vi "_getInfoForWfmGeneration.vi"(11 "Analysis State":T1) -> (1 "wfm info":cluster{i32, "variant":variant}[](array[cluster]), 3 "number of channels":i32)   [LabVIEW 2017]
uses:
  <vilib>/addons/InsightCM/Utilities/Analysis/Shared/controls/AnalysisSensorType.ctl
  <vilib>/addons/InsightCM/Utilities/Analysis/Shared/controls/AnalysisConversionOp.ctl
  <vilib>/addons/InsightCM/Utilities/Analysis/Shared/controls/AnalysisBandDomain.ctl
  <vilib>/addons/InsightCM/Utilities/Analysis/Shared/controls/AnalysisFeature.ctl
  <vilib>/addons/InsightCM/Utilities/Analysis/Shared/controls/AnalysisDynamicChannel.ctl
  <vilib>/addons/InsightCM/Utilities/Analysis/Shared/controls/AnalysisCalculatedMeasurementType.ctl
  <vilib>/addons/InsightCM/Utilities/Analysis/Shared/controls/AnalysisBandAmplitudeScale.ctl
  <vilib>/addons/InsightCM/Utilities/Analysis/Shared/controls/AnalysisBandCalculation.ctl
  <vilib>/addons/InsightCM/Utilities/Analysis/Shared/controls/AnalysisStaticChannel.ctl
  <vilib>/addons/InsightCM/Utilities/Analysis/Shared/controls/AnalysisDevice.ctl
  <vilib>/addons/InsightCM/Utilities/Analysis/Shared/controls/AnalysisSpeedProfile.ctl
  <vilib>/addons/InsightCM/Utilities/Analysis/Shared/controls/AnalysisState.ctl
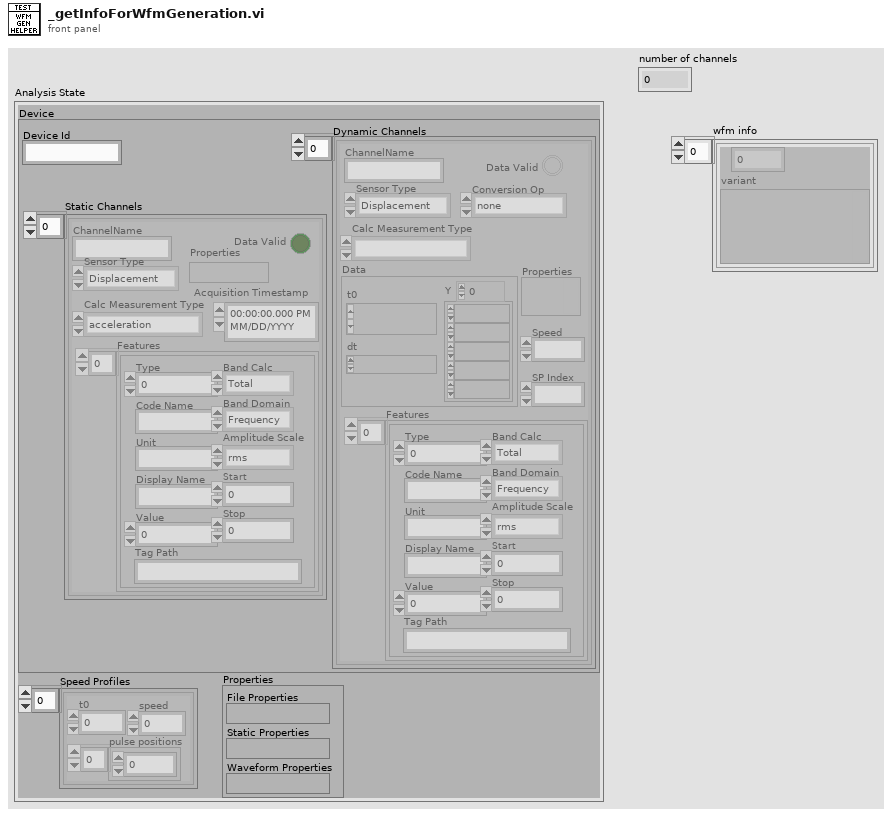
[diagram p1: front panel]
types:
  T1 = typedef "AnalysisState.ctl" = cluster{"Properties":cluster{"File Properties":variant, "Static Properties":variant, "Waveform Properties":variant}, "Properties Initialized?":bool, "Device":T2, "Speed Profiles":T12[]}
  T2 = typedef "AnalysisDevice.ctl" = cluster{"Device Id":string, "Dynamic Channels":T3[], "Static Channels":T11[]}
  T3 = typedef "AnalysisDynamicChannel.ctl" = cluster{"ChannelName":string, "Sensor Type":T4, "Conversion Op":T5, "Features":T6[], "Data":waveform(sgl), "Speed":sgl, "SP Index":i32, "Properties":variant, "Data Valid":bool, "Calc Measurement Type":T10}
  T4 = typedef "AnalysisSensorType.ctl" = enum16{"Accelerometer", "Velocity", "Displacement", "Tachometer", "Tempertature ", "dynamicVoltage", "Voltage", "Current", "Microphone", "Resistance", "Digital Input", "<Unknown>"}
  T5 = typedef "AnalysisConversionOp.ctl" = enum16{"none", "singleInt", "doubleInt", "singleDiff", "doubleDiff"}
  T6 = typedef "AnalysisFeature.ctl" = cluster{"Type":i32, "Code Name":string, "Unit":string, "Display Name":string, "Value":sgl, "Start":dbl, "Stop":dbl, "Band Domain":T7, "Band Calc":T8, "Amplitude Scale":T9, "Tag Path":string}
  T7 = typedef "AnalysisBandDomain.ctl" = enum16{"Frequency", "CPM", "Orders"}
  T8 = typedef "AnalysisBandCalculation.ctl" = enum16{"Total", "Max", "Phase"}
  T9 = typedef "AnalysisBandAmplitudeScale.ctl" = enum16{"rms", "peak", "pk-pk", "phase", "<none>"}
  T10 = typedef "AnalysisCalculatedMeasurementType.ctl" = enum16{"acceleration", "velocity", "displacement", "tachometer", "speed", "temperature", "voltage", "current", "resistance", "digitalInput", "<Unknown>"}
  T11 = typedef "AnalysisStaticChannel.ctl" = cluster{"ChannelName":string, "Sensor Type":T4, "Features":T6[], "Properties":variant, "Data Valid":bool, "Calc Measurement Type":T10, "Acquisition Timestamp":timestamp}
  T12 = typedef "AnalysisSpeedProfile.ctl" = cluster{"t0":dbl, "pulse positions":sgl[], "speed":dbl}
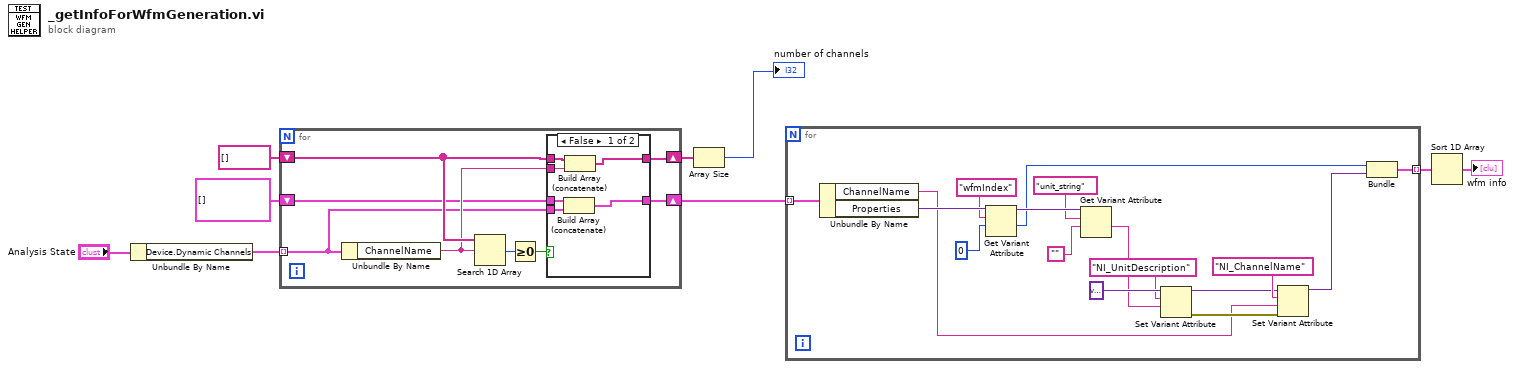
[diagram p0: block diagram]
diagram:
  n1 = Unbundle By Name("Analysis State") -> ("Device.Dynamic Channels"=w7:T3[])
  n2 = for {
    shift-right: [w14] -> w4
    shift-left: string[] [] -> [w15]
    tunnel: w7 -> [w12] mode=indexing
    shift-right: [w11] -> w3
    shift-left: T3[] [] -> [w10]
    n3 = Unbundle By Name(w12) -> ("ChannelName"=w13:string)
    n4 = Search 1D Array(1D array=w15, element=w13) -> (index of element=w16:i32)  [unwired: 1 in]
    n5 = Greater Or Equal To 0?(x=w16) -> (x >= 0?=w17:bool)
    n6 = case shown="False" w17 {
      tunnel: w15 -> [w23 w25]
      tunnel: [w22 w25] -> w14
      tunnel: w13 -> [w21 _]
      tunnel: w12 -> [w20 _]
      tunnel: [w19 w24] -> w11
      tunnel: w10 -> [w18 w24]
      frame False {
        n7 = Build Array (concatenate)(w18, w20) -> (w19:T3[])
        n8 = Build Array (concatenate)(w23, w21) -> (w22:string[])
      }
      frame True {
      }
    }
  }
  n9 = Array Size(array=w4) -> (size(s)=→"number of channels":i32)
  n10 = for {
    tunnel: w3 -> [w42] mode=indexing
    tunnel: [w26] -> w2 mode=indexing
    n11 = Unbundle By Name(w42) -> ("ChannelName"=w29:string, "Properties"=w41:variant)
    n12 = Get Variant Attribute(Variant=w41, name="wfmIndex", default value (empty Variant)=0) -> (duplicate Variant=w40:variant, value=w28:i32)  [unwired: 1 in, 2 out]
    n13 = Get Variant Attribute(Variant=w40, name="unit_string", default value (empty Variant)="") -> (value=w34:string)  [unwired: 1 in, 3 out]
    n14 = Set Variant Attribute(Variant=variant ("variant"), name="NI_UnitDescription", value=w34) -> (Variant out=w31:variant, error out=w30:errorcluster)  [unwired: 1 in, 1 out]
    n15 = Set Variant Attribute(Variant=w31, name="NI_ChannelName", value=w29, error in=w30) -> (Variant out=w27:variant)  [unwired: 2 out]
    n16 = Bundle(w28, "variant"=w27) -> (w26:cluster{i32, "variant":variant})  [unwired: 1 in]
  }
  n17 = Sort 1D Array(array=w2) -> (sorted array=→"wfm info":cluster{i32, "variant":variant}[])
